vi "Get all Measurement Service.vi"(8 "error in":errorcluster, 11 "Project ref":refnum<vi>) -> (0 "error out":errorcluster, 3 "Measurement Service Names":string[](array[string]))   [LabVIEW 2020, in "MeasurementService Editor.lvlib"]
uses:
  MeasurementService Editor.lvlib
  3e5c5311-854d-4fcf-ab0e-b2d0d29b1212.vi
  <vilib>/Comparison/Equal/Equal Functor/Equal Functor.lvclass
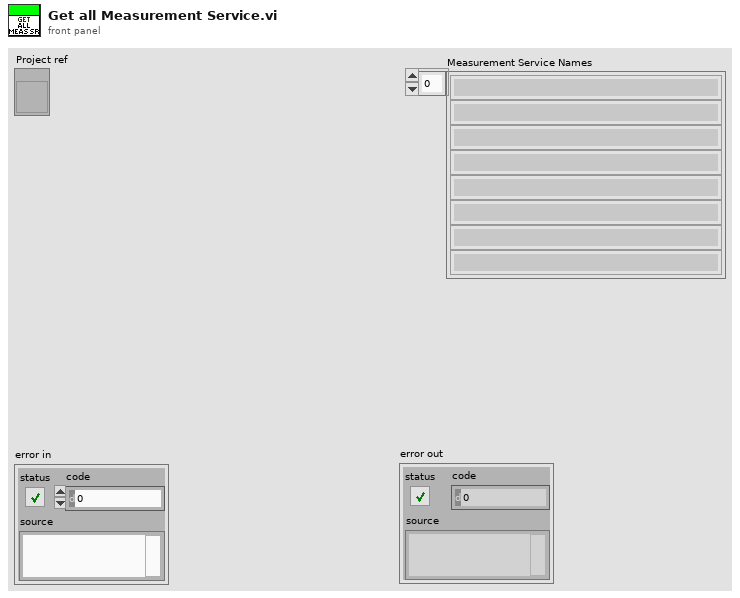
[diagram p1: front panel]
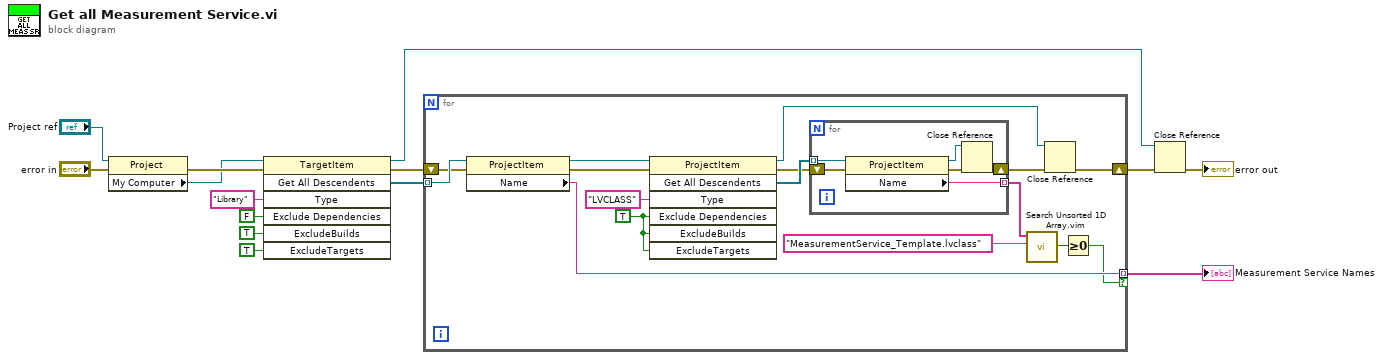
[diagram p0: block diagram]
diagram:
  n1 = property class="Project"(reference="Project ref", error in="error in") -> (error out=w8:errorcluster, "My Computer"=w7:refnum<vi>)  [unwired: 1 out]
  n2 = invoke class="TargetItem" method="Get All Descendents"(reference=w7, error in=w8, "Type"="Library", "Exclude Dependencies"=FALSE ("ExcludeDependencies"), "ExcludeBuilds"=TRUE, "ExcludeTargets"=TRUE) -> (reference out=w3:refnum<vi>, error out=w10:errorcluster, "All Descendents"=w11:refnum<vi>[])  [unwired: 1 in, 4 out]
  n3 = for {
    tunnel: w11 -> [w30] mode=indexing
    tunnel: [w29] -> w1 mode=indexing if=w17
    shift-right: [w27] -> w4
    shift-left: w10 -> [w28]
    w23 = TRUE ("ExcludeDependencies")
    n4 = property class="ProjectItem"(reference=w30, error in=w28) -> (reference out=w26:refnum<vi>, error out=w25:errorcluster, "Name"=w29:string)
    n5 = invoke class="ProjectItem" method="Get All Descendents"(reference=w26, error in=w25, "Type"="LVCLASS", "Exclude Dependencies"=w23, "ExcludeBuilds"=w23, "ExcludeTargets"=w23) -> (reference out=w24:refnum<vi>, error out=w15:errorcluster, "All Descendents"=w21:refnum<vi>[])  [unwired: 1 in, 4 out]
    n6 = for {
      tunnel: w21 -> [w36] mode=indexing
      tunnel: [w35] -> w20 mode=indexing
      shift-right: [w32] -> w16
      shift-left: w15 -> [w31]
      n7 = property class="ProjectItem"(reference=w36, error in=w31) -> (reference out=w34:refnum<vi>, error out=w33:errorcluster, "Name"=w35:string)
      n8 = Close Reference(reference=w34, error in (no error)=w33) -> (error out=w32:errorcluster)
    }
    n9 = call "Search Unsorted 1D Array.vim"("element"="MeasurementService_Template.lvclass", "unsorted 1D array"=w20) -> ("index of element"=w18:i32)  [unwired: 9 in]
    n10 = Close Reference(reference=w24, error in (no error)=w16) -> (error out=w27:errorcluster)
    n11 = Greater Or Equal To 0?(x=w18) -> (x >= 0?=w17:bool)
  }
  "Measurement Service Names" <- w1
  n12 = Close Reference(reference=w3, error in (no error)=w4) -> (error out=→"error out":errorcluster)
